vi "ALL_TEMPERATURE.vi"(11 "Numeric":i8) -> (3 "F":dbl)   [LabVIEW 2017]
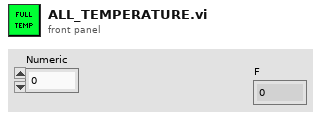
[diagram p1: front panel]
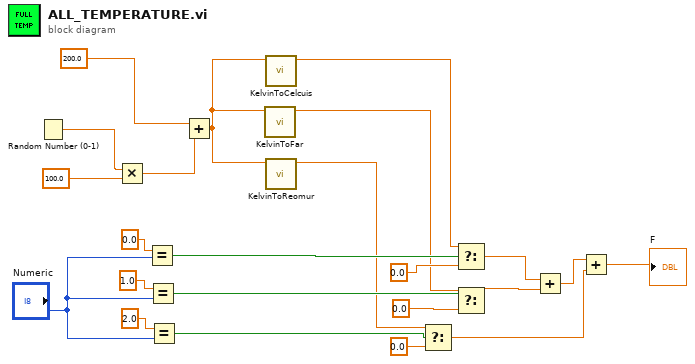
[diagram p0: block diagram]
diagram:
  n1 = Random Number (0-1) ("Random Number (200-300)")() -> (number: 0 to 1=w21:dbl)
  n2 = Multiply(x=w21, y=100.0) -> (x*y=w22:dbl)
  n3 = Equal?(x=0.0, y="Numeric") -> (x = y?=w14:bool)
  n4 = Equal?(x=1.0, y="Numeric") -> (x = y?=w13:bool)
  n5 = Equal?(x=2.0, y="Numeric") -> (x = y?=w12:bool)
  n6 = Add(x=200.0, y=w22) -> (x+y=w19:dbl)
  n7 = call "KelvinToFar.vi"("Кельвин"=w19) -> ("Фаренгейт"=w7:dbl)  [unwired: 10 in]
  n8 = call "KelvinToCelcuis.vi"("Кельвин"=w19) -> ("Цельсий"=w8:dbl)  [unwired: 10 in]
  n9 = call "KelvinToReomur.vi"("Кельвин"=w19) -> ("Реомюр"=w6:dbl)  [unwired: 10 in]
  n10 = Select(t=w6, s=w12, f=0.0) -> (s? t:f=w2:dbl)
  n11 = Select(t=w8, s=w14, f=0.0) -> (s? t:f=w5:dbl)
  n12 = Select(t=w7, s=w13, f=0.0) -> (s? t:f=w4:dbl)
  n13 = Add(x=w5, y=w4) -> (x+y=w3:dbl)
  n14 = Add(x=w3, y=w2) -> (x+y=→"F":dbl)
